vi "WT-Controller-OL.vi"() -> ()   [LabVIEW 2017]
uses:
  <vilib>/Platform/TimedLoop/XDataNode/timing_clust.ctl
  <vilib>/Platform/TimedLoop/XDataNode/nitl_modes.ctl
  <vilib>/Platform/TimedLoop/XDataNode/wakeup.ctl
  <vilib>/DAQmx/read.llb/DAQmx Read (Analog 1D DBL NChan 1Samp).vi
  <vilib>/Analysis/baseanly.llb/Mean (DBL).vi
  <vilib>/DAQmx/miscellaneous.llb/DAQmx Fill In Error Info.vi
  <vilib>/platform/TimedLoop/XDataNode/XDataNode.xnode
  <vilib>/Platform/TimedLoop/XDataNode/XDNodeRunTimeDep.lvlib
  <vilib>/Analysis/NI_AALBase.lvlib
panel:
  out "DRAG Average (N)":dbl
  out "DRAG Average (N)":dbl(knob) scale=0.0..10.0
  out "Velocity (mph)":dbl format="%0.2f"
  out "Fan (A)":dbl format="%0.2f"
  out "Drag":dbl(graph)
  out "Boolean":bool
  in  "POWER":bool
  out "error out":errorcluster
  in  "Velocity (m/s)":dbl
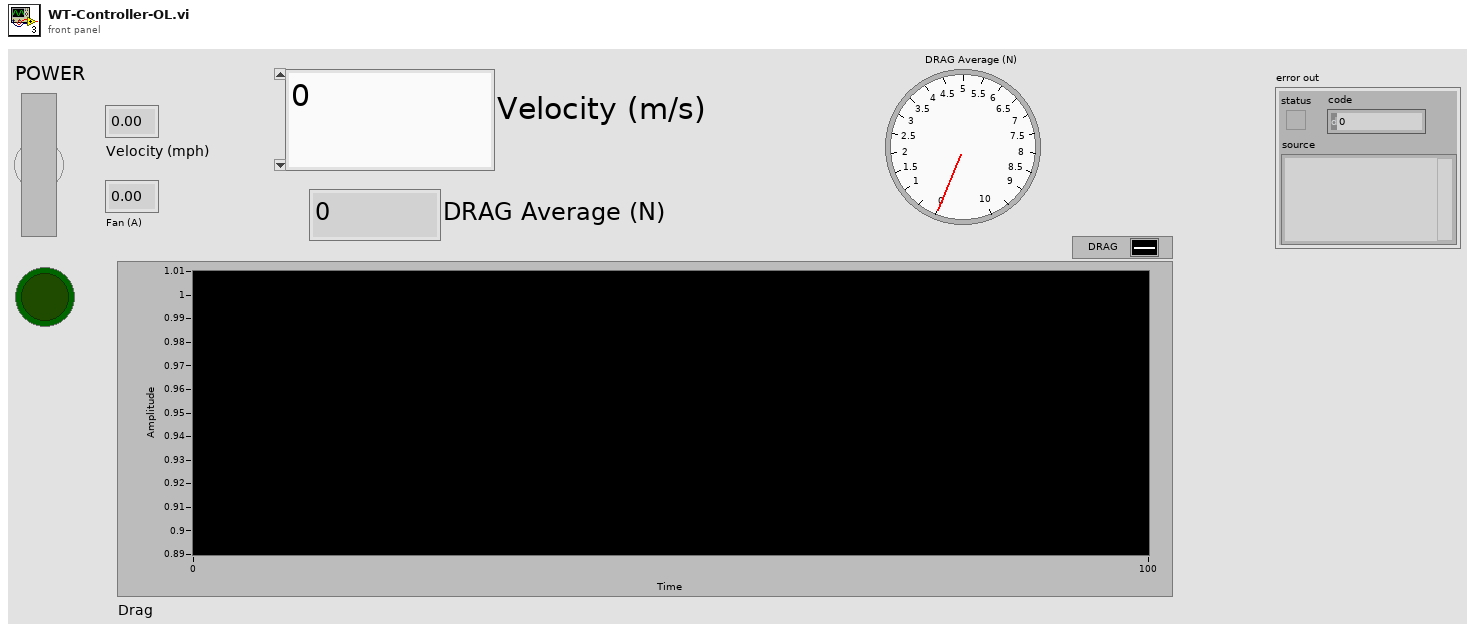
[diagram p1: front panel]
types:
  T1 = typedef "XDNodeRunTimeDep.lvlib/timing_clust.ctl" = cluster{"Expected End [f-1]":u64, "Actual End [f-1]":u64, "Finished Late? [f-1]":bool, "Expected End [i-1]":u64, "Actual End [i-1]":u64, "Finished Late? [i-1]":bool, "Expected Start [i]":u64, "Actual Start [i]":u64, "Expected Start [f]":u64, "Actual Start [f]":u64, "Source Name":string, "Structure Name":string, "Period":i64, "Deadline":i64, "Offset":i64, "Start":i64, "Priority":i32, "Timeout":i32, "Mode":T2, "Wakeup Reason":T3, "Error":errorcluster, "Source Type":string, "Secondary Source Type":string, "Global End Time":u64, "Global Start Time":u64, "Frame Duration":u64, "Iteration Duration":u64, "Assigned CPU":i32, "I/O Scan Engine Mode":u32}
  T2 = typedef "XDNodeRunTimeDep.lvlib/nitl_modes.ctl" = enum32{"No Change", "Process missed periods, maintain original phase", "Discard missed periods, maintain original phase", "Process missed periods, ignore original phase", "Discard missed periods, ignore original phase"}
  T3 = typedef "XDNodeRunTimeDep.lvlib/wakeup.ctl" = enum32{"Normal", "Aborted", "Asynchronous wakeup", "Timing source error", "Timed loop error", "Timeout"}
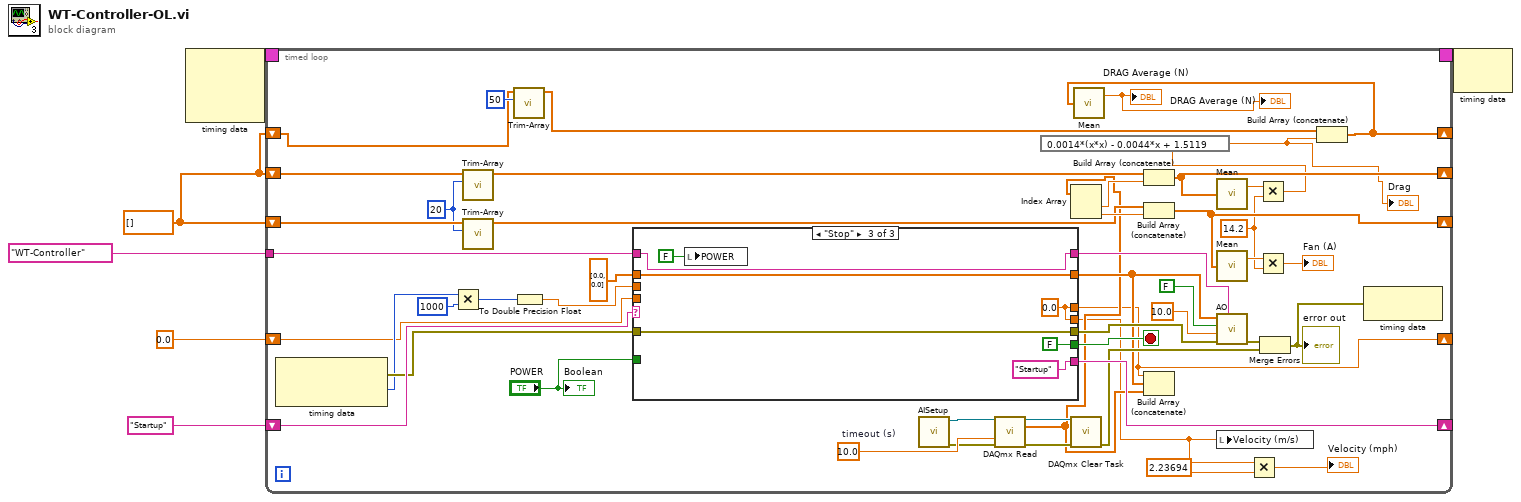
[diagram p0: block diagram]
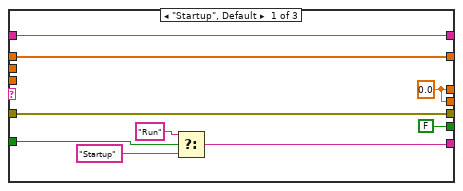
[diagram p2: hidden frame]
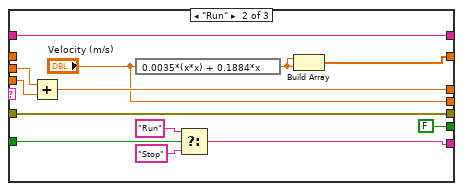
[diagram p3: hidden frame]
diagram:
  w1 = dbl[] []
  n1 = node-c288() -> (w4:T1)  [unwired: 3 in]
  n2 = timed-loop {
    shift-right: [w55] -> _
    shift-left: "Startup" -> [w56]
    tunnel: tag "WT-Controller" ("device name") -> [w53]
    timing: w4 -> [_]
    timing-out: [_] -> w3
    shift-right: [w34] -> _
    shift-left: w1 -> [w32]
    shift-right: [w33] -> _
    shift-left: w1 -> [w31]
    shift-right: [w17] -> _
    shift-left: 0.0 -> [w19]
    shift-right: [w9] -> _
    shift-left: w1 -> [w11]
    stop <- w54 stop-if-true
    w26 = 14.2 ("y")
    w29 = 20 ("length")
    w45 = 10.0  # timeout (s)
    n3 = node-c288() -> (w48:errorcluster, w22:i64)  [unwired: 1 in]
    n4 = Multiply(x=w22, y=i64 1000) -> (x*y=w20:i64)
    n5 = call "Trim-Array.vi"("length"=w29, "Array in"=w32) -> ("Array out"=w36:dbl[])  [unwired: 9 in]
    n6 = call "Trim-Array.vi"("length"=w29, "Array in"=w31) -> ("Array out"=w30:dbl[])  [unwired: 9 in]
    n7 = call "Trim-Array.vi"("length"=50, "Array in"=w11) -> ("Array out"=w12:dbl[])  [unwired: 9 in]
    n8 = To Double Precision Float(number=w20) -> (double precision float=w18:dbl)
    n9 = case shown="\"Stop\"" w56 {
      tunnel: [w65 w84 "Startup" ("f")] -> w55
      tunnel: [w70 w82 w89] -> w24
      tunnel: [FALSE ("Stop") FALSE ("Stop") FALSE ("Stop")] -> w54
      tunnel: w53 -> [w69 w81 w90]
      tunnel: [w71 w80 w88] -> w50
      tunnel: w48 -> [w71 w80 w88]
      tunnel: dbl[] [0.0, 0.0] ("appended array") -> [w70 _ w89]
      tunnel: [w69 w81 w90] -> w49
      tunnel: "POWER" -> [w67 w79 _]
      tunnel: w19 -> [_ w76 _]
      tunnel: [w63 w74 w85] -> w17
      tunnel: w18 -> [_ w75 _]
      tunnel: [w63 "Velocity (m/s)" w85] -> w16
      frame "Startup", Default {
        w63 = 0.0
        n10 = Select(t="Run" ("f"), s=w67, f="Startup") -> (s? t:f=w65:string)
      }
      frame "Run" {
        n11 = Add(x=w75, y=w76) -> (x+y=w74:dbl)
        n12 = expression code="0.0035*(x*x) + 0.1884*x"("Velocity (m/s)") -> (w73:dbl)
        n13 = Select(t="Run" ("f"), s=w79, f="Stop") -> (s? t:f=w84:string)
        n14 = Build Array(w73, w73) -> (w82:dbl[])
      }
      frame "Stop" {
        w85 = 0.0
        n15 = local write "POWER"(FALSE ("POWER")) -> ()
      }
    }
    n16 = call "AISetup.vi"() -> ("error out"=w41:errorcluster, "task out"=w42:refnum<k21>)  [unwired: 10 in]
    n17 = call-poly <vilib>:"DAQmx Read.vi"("task/channels in"=w42, "timeout"=w45, "error in"=w41) -> ("task out"=w43:refnum<k21>, "data"=w23:dbl[], "error out"=w44:errorcluster)  [unwired: 10 in]
    n18 = Index Array(array=w23) -> (element #1=w37:dbl, element #2=w35:dbl)  [unwired: 2 in]
    n19 = call <vilib>:"DAQmx Clear Task.vi"("task in"=w43, "error in"=w44) -> ("error out"=w40:errorcluster)  [unwired: 13 in]
    n20 = Build Array (concatenate)(w36, w37) -> (w34:dbl[])
    n21 = Build Array (concatenate)(w30, w35) -> (w33:dbl[])
    n22 = Build Array (concatenate)(w17, w24, w23) -> ()  [unwired: 1 out]
    n23 = call-poly <vilib>:"Mean.vi"("X"=w34) -> ("mean"=w28:dbl)  [unwired: 1 out]
    n24 = call-poly <vilib>:"Mean.vi"("X"=w33) -> ("mean"=w27:dbl)  [unwired: 1 out]
    n25 = call "AO.vi"("device name"=w49, "error in"=w50, "timeout (s)"=10.0, "stop (T)"=FALSE, "data"=w24) -> ("error out"=w39:errorcluster)  [unwired: 2 in, 1 out]
    n26 = local write "Velocity (m/s)"(w16) -> ()
    n27 = Multiply(x=w16, y=2.23694) -> (x*y=→"Velocity (mph)":dbl)
    n28 = Multiply(x=w28, y=w26) -> (x*y=w8:dbl)
    n29 = expression code="0.0014*(x*x) - 0.0044*x + 1.5119"(w8) -> (w7:dbl)
    "Drag" <- w7
    n30 = Multiply(x=w27, y=w26) -> (x*y=→"Fan (A)":dbl)
    n31 = Merge Errors(w39, w40) -> (w38:errorcluster)
    "error out" <- w38
    n32 = Build Array (concatenate)(w12, w7) -> (w9:dbl[])
    n33 = call-poly <vilib>:"Mean.vi"("X"=w9) -> ("mean"=→"DRAG Average (N)" →"DRAG Average (N)":dbl)  [unwired: 1 out]
    n34 = node-c288(w38) -> ()  [unwired: 1 out]
    "Boolean" <- "POWER"
  }
  n35 = node-c288(w3) -> ()  [unwired: 1 out]
